vi "getResults.vi"(8 "error in (no error)":errorcluster, 11 "AbsorptionAnalyser in":refnum<class "AbsorptionAnalyser.lvclass">) -> (0 "error out":errorcluster, 2 "results":T1, 3 "AbsorptionAnalyser out":refnum<class "AbsorptionAnalyser.lvclass">)   [LabVIEW 2009, in "Tools.lvlib" / "Imaging.lvlib" / "AbsorptionAnalyser.lvclass"]
uses:
  AbsorptionAnalyser.lvclass
  AbsorptionAnalyser.lvclass/AbsorptionAnalyser.ctl
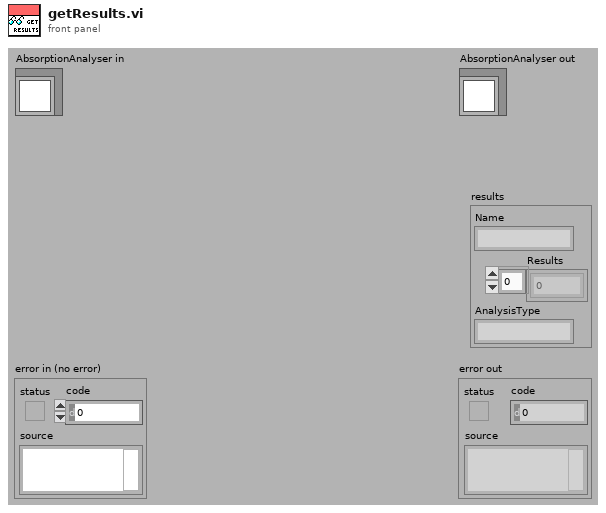
[diagram p1: front panel]
types:
  T1 = cluster{"Name":string, "Results":dbl[], "AnalysisType":string}
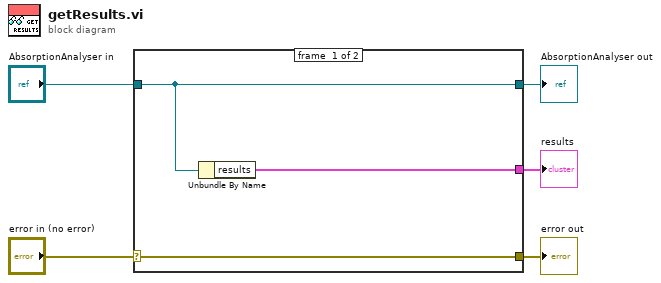
[diagram p0: block diagram]
diagram:
  n1 = case shown="No Error" "error in (no error)" {
    selector: "error in (no error)" -> [w8 w9]
    tunnel: [w8 w9] -> w4
    tunnel: [w7 w10] -> w2
    tunnel: "AbsorptionAnalyser in" -> [w7 w10]
    tunnel: [w6 _] -> w1
    frame #0 {
      n2 = Unbundle By Name(w7) -> ("results"=w6:T1)
    }
    frame #1 {
    }
  }
  "error out" <- w4
  "AbsorptionAnalyser out" <- w2
  "results" <- w1
